vi "Rollback Transaction on Error.vi"(7 "error in":errorcluster, 10 "Connection In":refnum<k7>) -> (0 "error out":errorcluster, 3 "Connection Out":refnum<k7>)   [LabVIEW 2022 SP3, in "hse-db-ado.lvlib" / "ADO-DB-Driver.lvlib"]
doc: "Rollback the transaction\n\n____\nHAMPEL SOFTWARE ENGINEERING v1.4.0 (2023-12-19 09:52)"
uses:
  ADO-DB-Driver.lvlib
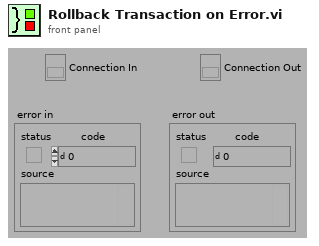
[diagram p1: front panel]
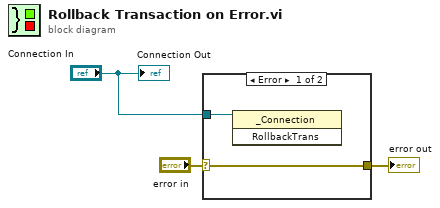
[diagram p0: block diagram]
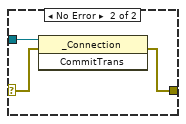
[diagram p2: hidden frame]
diagram:
  n1 = case shown="Error" "error in" {
    selector: "error in" -> [w4 w7]
    tunnel: [w4 w6] -> w2
    tunnel: "Connection In" -> [w5 w8]
    frame Error {
      n2 = invoke class="_Connection" method="RollbackTrans"(reference=w5) -> ()  [unwired: 2 in, 3 out]
    }
    frame No Error {
      n3 = invoke class="_Connection" method="CommitTrans"(reference=w8, error in=w7) -> (error out=w6:errorcluster)  [unwired: 1 in, 2 out]
    }
  }
  "error out" <- w2
  "Connection Out" <- "Connection In"
